vi "GetFileAttributes.vi"() -> ()   [LabVIEW 2011]
uses:
  kernel32.dll
panel:
  out "error out":errorcluster
  in  "error in (no error)":errorcluster
  out "File Attributes":cluster{bool, bool, bool, bool, bool, bool}
  in  "FileName":string
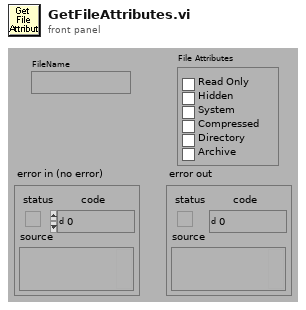
[diagram p1: front panel]
types:
  T1 = cluster{"Boolean array[0]":bool, "Boolean array[1]":bool, "Boolean array[2]":bool, "Boolean array[3]":bool, "Boolean array[4]":bool, "Boolean array[5]":bool}
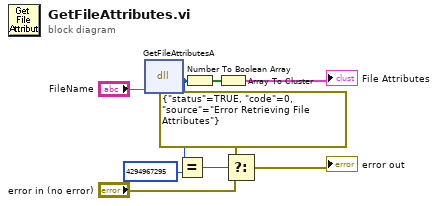
[diagram p0: block diagram]
diagram:
  n1 = dll-call lib="kernel32.dll" fn="GetFileAttributesA"("lpFileName"="FileName") -> (w6:u32)  [unwired: 4 in, 2 out]
  n2 = Equal?(x=w6, y=u32 4294967295) -> (x = y?=w4:bool)
  n3 = Number To Boolean Array(number=w6) -> (Boolean array=w8:bool[])
  n4 = Array To Cluster(array=w8) -> (cluster=→"File Attributes":T1)
  n5 = Select(t=errorcluster {"status"=TRUE, "code"=0, "source"="Error Retrieving File Attributes"}, s=w4, f="error in (no error)") -> (s? t:f=→"error out":errorcluster)
